vi "Array FIFO（DBL）.vi"(7 "init":bool caption="初始化", 10 "length":i32=100 caption="采样长度", 11 "input":dbl caption="输入数据点" format="%0.2f") -> (1 "Previous Queue":dbl[](array[numeric]) caption="之前队列", 2 "Current Queue":dbl[](array[numeric]) caption="当前队列", 3 "eliminated":dbl caption="已除去的元素" format="%0.2f", 4 "current length":i32 caption="当前长度")   [LabVIEW 2012, in "Array FIFO.lvlib"]
uses:
  Array FIFO.lvlib
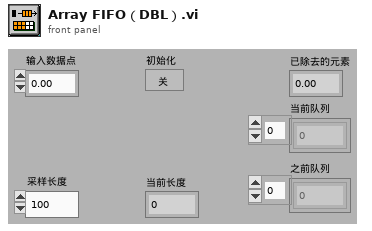
[diagram p1: front panel]
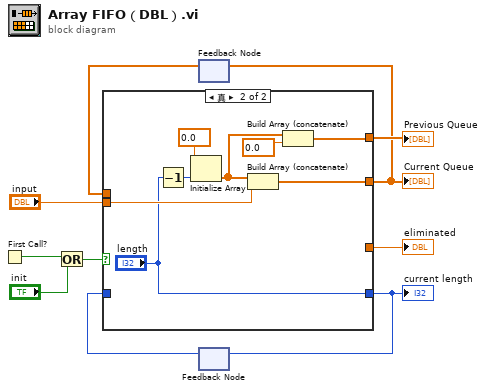
[diagram p0: block diagram]
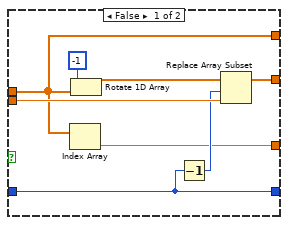
[diagram p2: hidden frame]
diagram:
  n1 = First Call?() -> (First Call?: T/F=w4:bool)
  n2 = Or(x=w4, y="init") -> (x .or. y?=w5:bool)
  n3 = feedback #1() -> (w8:dbl[])  [unwired: 1 in]
  n4 = feedback #2() -> (w9:i32)  [unwired: 1 in]
  n5 = case shown="真" w5 {
    tunnel: [w16 w20] -> w3
    tunnel: [w13 "length"] -> w2
    tunnel: w9 -> [w13 _]
    tunnel: w8 -> [w14 _]
    tunnel: "input" -> [w17 w26]
    tunnel: [w14 w21] -> w10
    tunnel: [w11 _] -> w1
    frame False {
      n6 = Index Array(array=w14) -> (element=w11:dbl)  [unwired: 1 in]
      n7 = Rotate 1D Array(1:w14, 2:i16 -1 ("n")) -> (0:w15:dbl[])
      n8 = Decrement(x=w13) -> (x-1=w12:i32)
      n9 = Replace Array Subset(array=w15, new element=w17, index=w12) -> (w16:dbl[])
    }
    frame True {
      n10 = Decrement(x="length") -> (x-1=w25:i32)
      n11 = Initialize Array(0.0 ("Element Data"), w25) -> (w23:dbl[])
      n12 = Build Array (concatenate)(w23, w26) -> (w20:dbl[])
      n13 = Build Array (concatenate)(w23, 0.0 ("Input Element")) -> (w21:dbl[])
    }
  }
  "Current Queue" <- w3
  "current length" <- w2
  "Previous Queue" <- w10
  "eliminated" <- w1
  n14 = feedback-in #1(w3) -> ()
  n15 = feedback-in #2(w2) -> ()
